vi "Get PID Paras.vi"(8 "error in (no error)":errorcluster, 11 "SGDV_Ctrl_Class in":refnum<class "SGDV Motor.lvclass">) -> (0 "error out":errorcluster, 2 "PID Paras":T1={"Output Range(deg/s)"={"output high"=720.0, "output low"=-720.0}, "PID gains"={"proportional gain (Kc)"=6.5, "integral time (Ti, min)"=0.0075, "derivative time (Td, min)"=0.0005}} {"PID gains"."derivative time (Td, min)" format="%.4f"; "PID gains"."integral time (Ti, min)" format="%.4f"; "PID gains"."proportional gain (Kc)" format="%.4f"; "Output Range(deg/s)"."output low" format="%.2f"; "Output Range(deg/s)"."output high" format="%.2f"}, 3 "SGDV_Ctrl_Class out":refnum<class "SGDV Motor.lvclass">)   [LabVIEW 2013, in "SGDV_Ctrl_v13_lib.lvlib" / "SGDV Motor.lvclass"]
uses:
  SGDV Motor.lvclass
  Controls and General VIs/PID Paras.ctl
  SGDV Motor.lvclass/SGDV Motor.ctl
  SGDV_Ctrl_v13_lib.lvlib
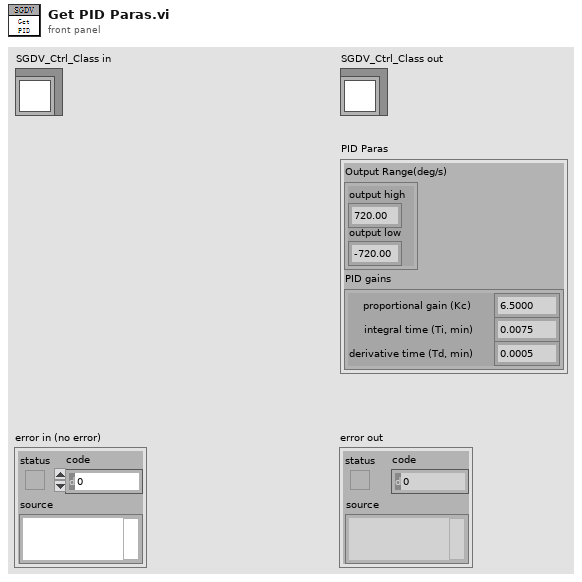
[diagram p1: front panel]
types:
  T1 = typedef "SGDV_Ctrl_v13_lib.lvlib/PID Paras.ctl" = cluster{"Output Range(deg/s)":cluster{"output high":dbl, "output low":dbl}, "PID gains":cluster{"proportional gain (Kc)":dbl, "integral time (Ti, min)":dbl, "derivative time (Td, min)":dbl}}
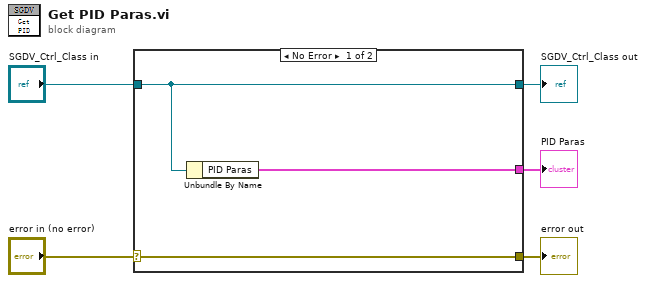
[diagram p0: block diagram]
diagram:
  n1 = case shown="No Error" "error in (no error)" {
    selector: "error in (no error)" -> [w8 w9]
    tunnel: [w8 w9] -> w4
    tunnel: [w7 w10] -> w2
    tunnel: "SGDV_Ctrl_Class in" -> [w7 w10]
    tunnel: [w6 _] -> w1
    frame No Error {
      n2 = Unbundle By Name(w7) -> ("PID Paras"=w6:T1)
    }
    frame Error {
    }
  }
  "error out" <- w4
  "SGDV_Ctrl_Class out" <- w2
  "PID Paras" <- w1
